vi "Do.vi"(8 "error in (no error)":errorcluster, 10 "Actor in":refnum<class "Actor.lvclass">, 11 "Acquire data class":refnum<class "Acquire data msg.lvclass">) -> (0 "error out":errorcluster, 2 "Actor out":refnum<class "Actor.lvclass">)   [LabVIEW 2015, in "Acquire data msg.lvclass"]
doc: "(<B>Filename</B>: Actor Framework.lvlib:Message.lvclass:Do.vi)\n\nDefines what a message does when it is received by an actor. Generally, a message instructs an actor to invoke one of its methods. By default, this method does nothing. A child class must override it to define behavior. Create a child class by using the Actor Framework Message Maker dialog box."
uses:
  Acquire data msg.lvclass
  <vilib>/ActorFramework/Actor/Actor.lvclass
  Gage digitizer actor.lvclass
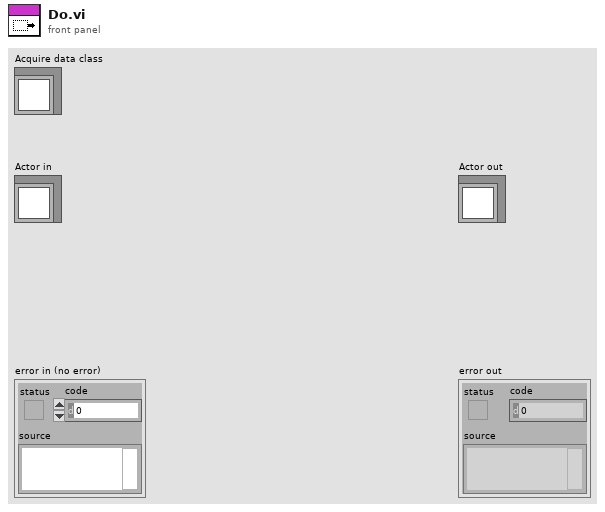
[diagram p1: front panel]
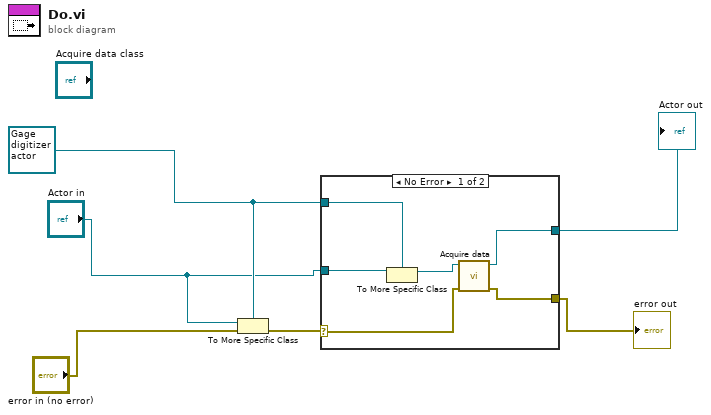
[diagram p0: block diagram]
diagram:
  w3 = refnum<class "Gage digitizer actor.lvclass"> refnum ("Gage digitizer actor.lvclass")
  n1 = To More Specific Class(target class=w3, reference="Actor in", error in="error in (no error)") -> (error out=w1:errorcluster)  [unwired: 1 out]
  n2 = case shown="No Error" w1 {
    selector: w1 -> [w10 w14]
    tunnel: "Actor in" -> [w12 w13]
    tunnel: [w7 w14] -> w6
    tunnel: w3 -> [w11 _]
    tunnel: [w8 w13] -> w4
    frame No Error {
      n3 = To More Specific Class(target class=w11, reference=w12) -> (specific class reference=w9:refnum<class "Gage digitizer actor.lvclass">)  [unwired: 1 in, 1 out]
      n4 = call-dynamic "Acquire data.vi"("error in (no error)"=w10, "Gage digitizer actor in"=w9) -> ("error out"=w7:errorcluster, "Gage digitizer actor out"=w8:refnum<class "Gage digitizer actor.lvclass">)  [unwired: 8 in]
    }
    frame Error {
    }
  }
  "error out" <- w6
  "Actor out" <- w4
